vi "Add Message.vi"(0 "TimeStamper in":refnum<class "TimeStamper.lvclass">, 5 "Channel":u8, 7 "Message":string, 9 "Time Stamp":timestamp, 11 "error in (no error)":errorcluster) -> (4 "TimeStamper out":refnum<class "TimeStamper.lvclass">, 6 "Cluster":T1, 15 "error out":errorcluster)   [LabVIEW 2014, in "TimeStamper.lvclass"]
uses:
  TimeStamper.lvclass
  TimeStamper.lvclass/TimeStamper.ctl
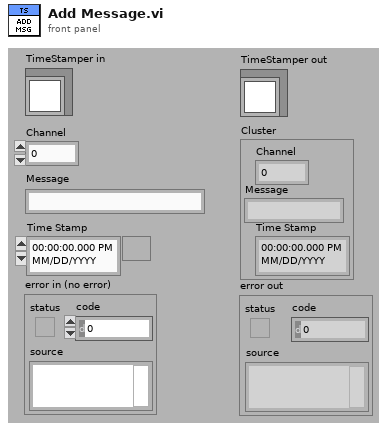
[diagram p1: front panel]
types:
  T1 = cluster{"Channel":u8, "Message":string, "Time Stamp":timestamp}
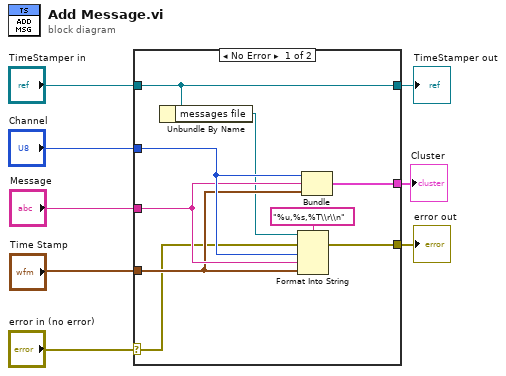
[diagram p0: block diagram]
diagram:
  n1 = case shown="No Error" "error in (no error)" {
    selector: "error in (no error)" -> [w11 w19]
    tunnel: [w10 w19] -> w7
    tunnel: [w13 w18] -> w5
    tunnel: "TimeStamper in" -> [w13 w18]
    tunnel: "Channel" -> [w16 _]
    tunnel: "Message" -> [w15 _]
    tunnel: "Time Stamp" -> [w14 _]
    tunnel: [w9 _] -> w1
    frame No Error {
      n2 = Unbundle By Name(w13) -> ("messages file"=w12:refnum<file>)
      n3 = Format Into String(format string="%u,%s,%T\\r\\n", initial string=w12, error in=w11, w16, w15, w14) -> (error out=w10:errorcluster)  [unwired: 1 out]
      n4 = Bundle("Channel"=w16, "Message"=w15, "Time Stamp"=w14) -> (w9:T1)  [unwired: 1 in]
    }
    frame Error {
    }
  }
  "error out" <- w7
  "TimeStamper out" <- w5
  "Cluster" <- w1
